vi "简单测试.vi"() -> ()   [LabVIEW 2014]
uses:
  <vilib>/Utility/NIReport.llb/image depth.ctl
  <vilib>/Utility/NIReport.llb/Append Report Text (str wrap).vi
  <vilib>/printing/ReportDocExtensions.llb/Append Front Panel Image to Report (refnum).vi
  <vilib>/Utility/NIReport.llb/NI_report.lvclass
  <vilib>/Utility/NIReport.llb/NI_ReportGenerationCore.lvlib
panel:
  out "波形图":dbl[](graph)
  in  "表格控件":string[][](table)
  in  "report file path":path caption="报表文件路径"
  in  "report type":T1(ring) caption="报表类型"
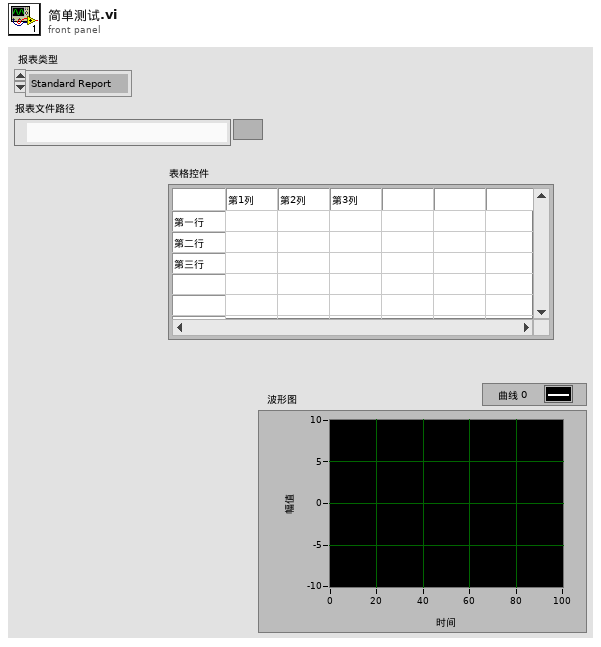
[diagram p1: front panel]
types:
  T1 = enum16{"Standard Report", "HTML", "Word", "Excel"}
  T2 = typedef "NI_ReportGenerationCore.lvlib/image depth.ctl" = u16
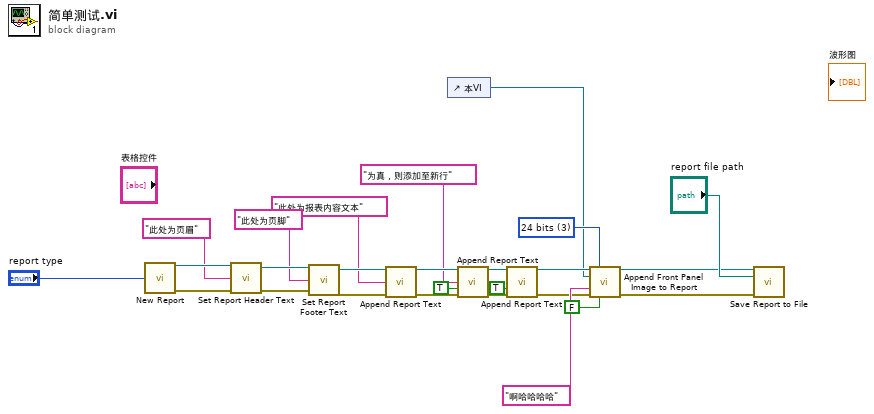
[diagram p0: block diagram]
diagram:
  w10 = T2 3 items=["B&W", "4 bits", "8 bits", "24 bits"] ("image depth")
  n1 = call <vilib>:"New Report.vi"("report type"="report type") -> ("report out"=w24:refnum<class "NI_report.lvclass">, "error out"=w25:errorcluster)  [unwired: 13 in]
  n2 = call-dynamic "Set Report Header Text.vi"("report in"=w24, "center header text"="此处为页眉", "error in (no error)"=w25) -> ("report out"=w21:refnum<class "NI_report.lvclass">, "error out"=w22:errorcluster)  [unwired: 11 in]
  n3 = call-dynamic "Set Report Footer Text.vi"("report in"=w21, "center footer text"="此处为页脚", "error in (no error)"=w22) -> ("report out"=w18:refnum<class "NI_report.lvclass">, "error out"=w19:errorcluster)  [unwired: 11 in]
  n4 = call-poly <vilib>:"Append Report Text.vi"("report in"=w18, "text"="此处为报表内容文本", "error in (no error)"=w19) -> ("report out"=w15:refnum<class "NI_report.lvclass">, "error out"=w16:errorcluster)  [unwired: 9 in, 2 out]
  n5 = control-ref of="本VI"() -> (w2:refnum<vi>)
  n6 = call-poly <vilib>:"Append Report Text.vi"("report in"=w15, "text"="为真，则添加至新行", "append on new line? (F)"=TRUE, "error in (no error)"=w16) -> ("report out"=w6:refnum<class "NI_report.lvclass">, "error out"=w7:errorcluster)  [unwired: 8 in, 2 out]
  n7 = call-poly <vilib>:"Append Report Text.vi"("report in"=w6, "append on new line? (F)"=TRUE, "error in (no error)"=w7) -> ("report out"=w3:refnum<class "NI_report.lvclass">, "error out"=w4:errorcluster)  [unwired: 9 in, 2 out]
  n8 = call-poly <vilib>:"Append Front Panel Image to Report.vi"("report in"=w3, "alignment (default)"=w10, "VI"=w2, "description"="啊哈哈哈哈", "error in (no error)"=w4, "visible area only?"=FALSE) -> ("report out"=w8:refnum<class "NI_report.lvclass">, "error out"=w9:errorcluster)  [unwired: 5 in, 3 out]
  n9 = call-dynamic "Save Report to File.vi"("report in"=w8, "report file path"="report file path", "error in (no error)"=w9) -> ()  [unwired: 11 in, 2 out]
